vi "WaveformToAIData.vi"(8 "error in (no error)":errorcluster, 10 "AI Channel":T1, 11 "AI Waveform":waveform(dbl)) -> (0 "error out":errorcluster, 3 "AI Data":T2)   [LabVIEW 2013, in "NI Card.lvclass"]
uses:
  NI Card.lvclass
  AI_Data.ctl
  <vilib>/Waveform/WDTOps.llb/WDT Get Waveform Time Array DBL.vi
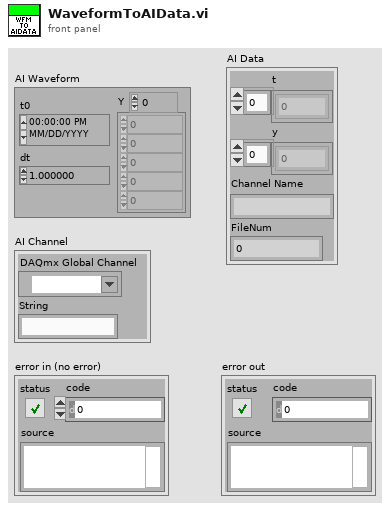
[diagram p1: front panel]
types:
  T1 = cluster{"DAQmx Global Channel":refnum<k21>, "String":string}
  T2 = typedef "NI Card.lvclass/AI_Data.ctl" = cluster{"t":dbl[], "y":dbl[], "Channel Name":string, "FileNum":u32}
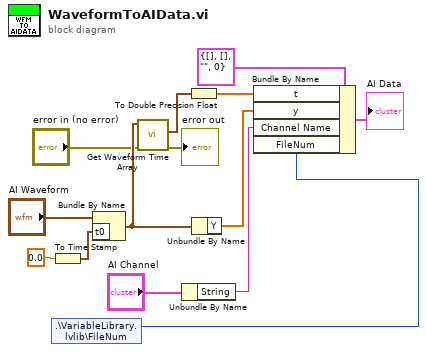
[diagram p0: block diagram]
diagram:
  n1 = shared-variable ".\\VariableLibrary.lvlib\\FileNum"() -> (w1:u32)  [unwired: 1 in, 1 out]
  n2 = To Time Stamp(1:0.0 ("number")) -> (0:w8:timestamp)
  n3 = Bundle By Name(cluster="AI Waveform", "t0"=w8) -> (w6:waveform(dbl))
  n4 = call-poly <vilib>:"Get Waveform Time Array.vi"("error in (no error)"="error in (no error)", "waveform in"=w6) -> ("error out"=→"error out":errorcluster, "X array"=w4:timestamp[])  [unwired: 8 out]
  n5 = Unbundle By Name("AI Channel") -> ("String"=w13:string)
  n6 = To Double Precision Float(number=w4) -> (double precision float=w12:dbl[])
  n7 = Unbundle By Name(w6) -> ("Y"=w11:dbl[])
  n8 = Bundle By Name(cluster=T2 {"t"=[], "y"=[], "Channel Name"="", "FileNum"=0} ("AI Data"), "t"=w12, "y"=w11, "Channel Name"=w13, "FileNum"=w1) -> (→"AI Data":T2)
